vi "error save.vi"(0 "file path (dialog if empty)":path, 1 "format (%.3f)":string="%.3f", 2 "Paramter guess":dbl[](array[numeric]), 5 "2D data":dbl[][](array[numeric]), 7 "1D data":dbl[](array[numeric]), 9 "append to file? (new file:F)":bool, 11 "error in (no error)":errorcluster, 12 "transpose? (no:F)":bool, 13 "delimiter (\\t)":string="\t") -> (4 "new file path (Not A Path if cancelled)":path, 15 "error out":errorcluster)   [LabVIEW 2018]
doc: "Converts a 2D or 1D array of strings, signed integers, or double-precision numbers to a text string and writes the string to a new byte stream file or appends the string to an existing file. Wire data to the <B>2D data</B> input or <B>1D data</B> input to determine the polymorphic instance to use or manually select the instance.\n\nUse this VI to transpose or separate data.\n\n<B>Note</B> To format with Microsoft Excel, use ActiveX with LabVIEW or the Report Generation Toolkit for Microsoft Office."
panel:
  in  "prompt":string="Choose file to write."
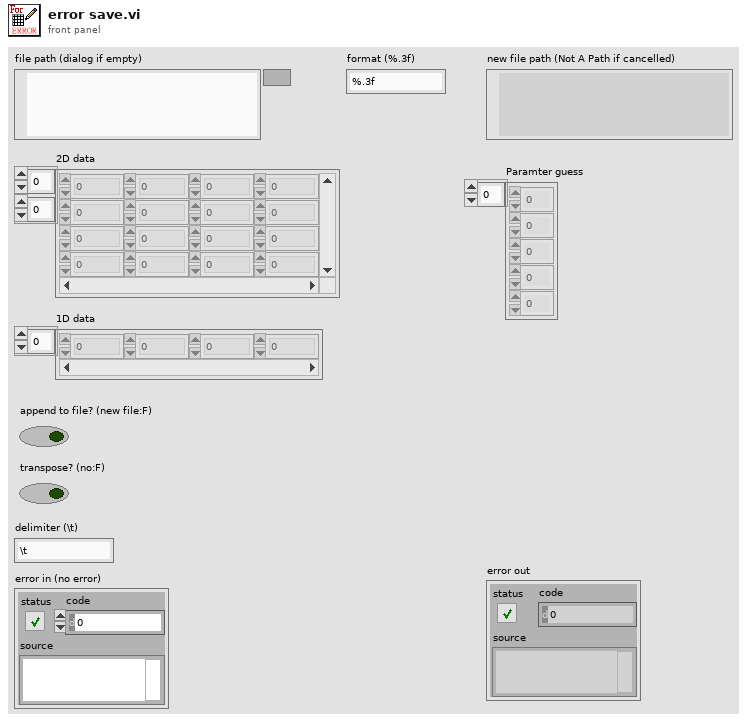
[diagram p1: front panel]
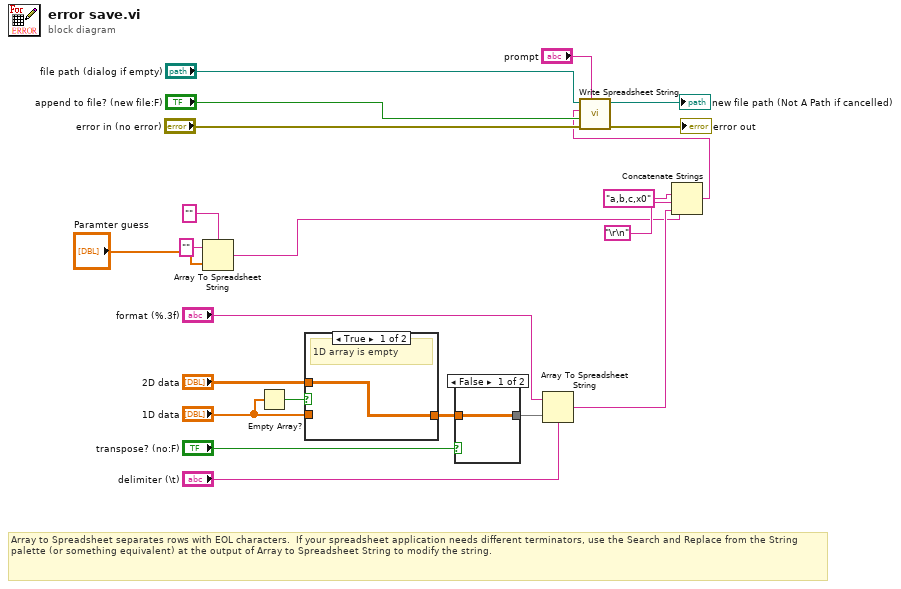
[diagram p0: block diagram]
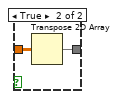
[diagram p2: hidden frame]
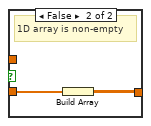
[diagram p3: hidden frame]
diagram:
  # "Array to Spreadsheet separates rows with EOL characters.  If your spreadsheet application needs different terminators, use the Search and Replace from the String palette (or something equivalent) at the output of Array to Spreadsheet String to modify the string."
  n1 = Array To Spreadsheet String(delimiter (Tab)="", array="Paramter guess", 3:"" ("format string")) -> (spreadsheet string=w3:string)
  n2 = Empty Array?(array="1D data") -> (empty?=w21:bool)
  n3 = case shown="True" w21 {
    tunnel: "1D data" -> [_ w25]
    tunnel: [w23 w24] -> w17
    tunnel: "2D data" -> [w23 _]
    frame True {
      # "1D array is empty"
    }
    frame False {
      # "1D array is non-empty"
      n4 = Build Array(w25) -> (w24:dbl[][])
    }
  }
  n5 = case shown="False" "transpose? (no:F)" {
    tunnel: [w26 w28] -> w15
    tunnel: w17 -> [w26 w27]
    frame False {
    }
    frame True {
      n6 = Transpose 2D Array(2D array=w27) -> (transposed array=w28:dbl[][])
    }
  }
  n7 = Array To Spreadsheet String(delimiter (Tab)="delimiter (\\t)", array=w15, 3:"format (%.3f)") -> (spreadsheet string=w6:string)
  n8 = Concatenate Strings(w3, "a,b,c,x0", "\r\n", w6) -> (w5:string)
  n9 = call <vilib>:"Write Spreadsheet String.vi"("prompt"="prompt", "error in"="error in (no error)", "append to file? (new file:F)"="append to file? (new file:F)", "spreadsheet string"=w5, "file path (dialog if empty)"="file path (dialog if empty)") -> ("error out"=→"error out":errorcluster, "path"=→"new file path (Not A Path if cancelled)":path)  [unwired: 5 in]
